vi "VI Data to JSON.vi"(7 "Port number":u16=3363, 8 "error in":errorcluster, 11 "VI Path":path) -> (0 "error out":errorcluster, 3 "JSON string":string)   [LabVIEW 2019]
uses:
  <vilib>/Utility/traverseref.llb/TRef TravTarget.ctl
  <vilib>/Utility/traverseref.llb/VI Scripting - Traverse.lvlib
  <vilib>/Utility/miscctls.llb/LVPositionTypeDef.ctl
  <vilib>/Utility/miscctls.llb/LVMapReplaceAction.ctl
  <vilib>/Utility/miscctls.llb/LVBoundsTypeDef.ctl
  Typedefs/FP Data.ctl
  Typedefs/BD Data.ctl
  Typedefs/VI Data.ctl
  Typedefs/VI Metadata.ctl
  Typedefs/Diagram Group.ctl
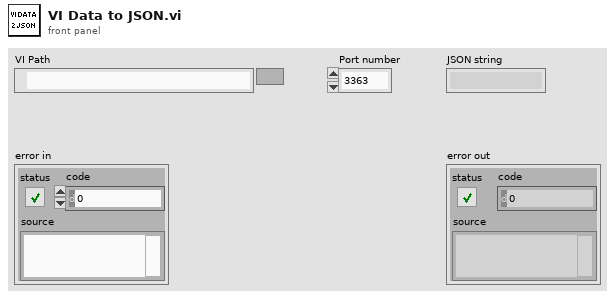
[diagram p1: front panel]
types:
  T1 = typedef "VI Data.ctl" = cluster{"Structure to Diagram":cluster{"UID":i32, "Diagram Group":T2}[], "Diagram to Structure":cluster{"Diagram UID":i32, "Diagram Children":i32[]}[], "FP":T5, "BD":T6, "Metadata":T7}
  T2 = typedef "Diagram Group.ctl" = cluster{"Diagram Data":cluster{"UID":i32, "Diagram Image":string}[], "Position":T3, "Bounds":T4, "Is on TLD?":bool, "Default Frame":u32}
  T3 = typedef "LVPositionTypeDef.ctl" = cluster{"Left":i32, "Top":i32}
  T4 = typedef "LVBoundsTypeDef.ctl" = cluster{"Width":u32, "Height":u32}
  T5 = typedef "FP Data.ctl" = cluster{"Bounds":T4, "Position":T3, "Color":string, "Image":string}
  T6 = typedef "BD Data.ctl" = cluster{"Bounds":T4, "Position":T3, "Color":string, "Image":string}
  T7 = typedef "VI Metadata.ctl" = cluster{"Image":string, "Description":string, "VI Name":string}
  T8 = typedef "imagedata.ctl" = cluster{"image type":i32, "image depth":i32, "image":u8[], "mask":u8[], "colors":u32[], "Rectangle":cluster{"left":i16, "top":i16, "right":i16, "bottom":i16}}
  T9 = typedef "TRef TravTarget.ctl" = enum16{"FP", "BD", "Other"}
  T10 = typedef "LVMapReplaceAction.ctl" = enum32{"Modify Entry only if found", "Add or Modify Entry", "Delete Entry"}
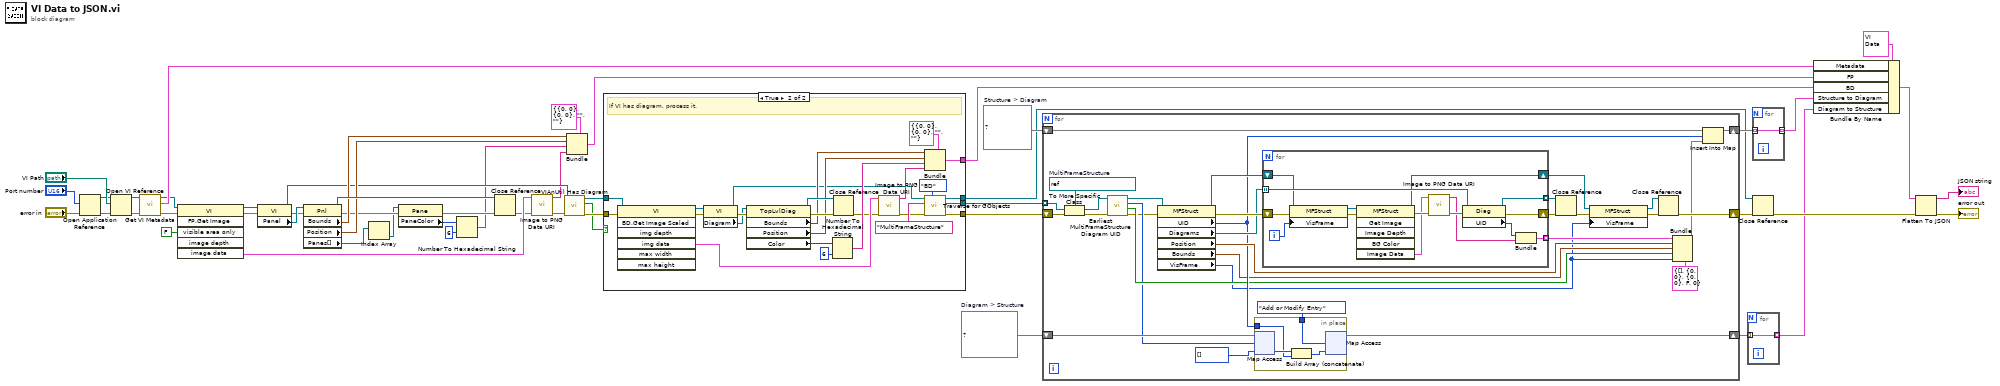
[diagram p0: block diagram]
diagram:
  w41 = map{i32, i32[]} {}  # Diagram > Structure
  w42 = map{i32, T2} {}  # Structure > Diagram
  n1 = Open Application Reference(8:"error in", 10:"Port number") -> (0:w40:errorcluster, 3:w38:refnum<vi>)  [unwired: 2 in]
  n2 = Open VI Reference(application reference (local)=w38, vi path="VI Path", error in (no error)=w40) -> (vi reference=w16:refnum<vi>, error out=w17:errorcluster)  [unwired: 3 in]
  n3 = call "Get VI Metadata.vi"("error in"=w17, "vi reference in"=w16) -> ("error out"=w15:errorcluster, "Metadata"=w14:T7, "vi reference out"=w9:refnum<vi>)  [unwired: 7 in]
  n4 = invoke class="VI" method="FP.Get Image"(reference=w9, error in=w15, "visible area only"=FALSE ("Visible Area Only")) -> (reference out=w34:refnum<vi>, error out=w33:errorcluster, "image data"=w25:T8)  [unwired: 3 in, 3 out]
  n5 = property class="VI"(reference=w34, error in=w33) -> (reference out=w24:refnum<vi>, error out=w35:errorcluster, "Panel"=w36:refnum<vi>)
  n6 = property class="Pnl"(reference=w36, error in=w35) -> (reference out=w32:refnum<vi>, error out=w7:errorcluster, "Bounds"=w31:T4, "Position"=w30:T3, "Panes[]"=w8:refnum<vi>[])
  n7 = Index Array(array=w8) -> (element=w5:refnum<vi>)  [unwired: 1 in]
  n8 = property class="Pane"(reference=w5, error in=w7) -> (error out=w6:errorcluster, "PaneColor"=w3:u32)  [unwired: 1 out]
  n9 = Number To Hexadecimal String(1:i16 6 ("width (-)"), 2:w3) -> (0:w1:string)
  n10 = Close Reference(reference=w32, error in (no error)=w6) -> (error out=w13:errorcluster)
  n11 = call "Image to PNG Data URI.vi"("error in (no error)"=w13, "Image data"=w25) -> ("error out"=w12:errorcluster, "Base64 encoded"=w2:string)  [unwired: 7 in, 1 out]
  n12 = call <vilib>:"VIAnUtil Has Diagram.vi"("error in (no error)"=w12, "VI in"=w24) -> ("error out"=w22:errorcluster, "Has Diag?"=w21:bool, "VI out"=w23:refnum<vi>)  [unwired: 4 in, 3 out]
  n13 = Bundle(cluster=T5 {"Bounds"={"Width"=0, "Height"=0}, "Position"={"Left"=0, "Top"=0}, "Color"="", "Image"=""} ("FP"), "Bounds"=w31, "Position"=w30, "Color"=w1, "Image"=w2) -> (w27:T5)
  n14 = case shown="True" w21 {
    tunnel: [w53 w57] -> w18
    tunnel: [_ w66] -> w28
    tunnel: w23 -> [w52 w63]
    tunnel: w22 -> [w53 w62]
    tunnel: [_ w58] -> w20
    tunnel: [w52 w56] -> w19
    frame False {
      # "If VI does not have diagram (global, control, etc...), skip.\nTool will then show the result as empty block diagram."
    }
    frame True {
      # "If VI has diagram, process it."
      n15 = invoke class="VI" method="BD.Get Image Scaled"(reference=w63, error in=w62) -> (reference out=w77:refnum<vi>, error out=w78:errorcluster, "img data"=w65:T8)  [unwired: 5 in, 4 out]
      n16 = property class="VI"(reference=w77, error in=w78) -> (reference out=w59:refnum<vi>, error out=w76:errorcluster, "Diagram"=w75:refnum<vi>)
      n17 = property class="TopLvlDiag"(reference=w75, error in=w76) -> (reference out=w73:refnum<vi>, error out=w74:errorcluster, "Bounds"=w69:T4, "Position"=w68:T3, "Color"=w71:u32)
      n18 = Number To Hexadecimal String(1:i16 6 ("width (-)"), 2:w71) -> (0:w67:string)
      n19 = Close Reference(reference=w73, error in (no error)=w74) -> (error out=w54:errorcluster)
      n20 = call "Image to PNG Data URI.vi"("error in (no error)"=w54, "Image data"=w65) -> ("error out"=w55:errorcluster, "Base64 encoded"=w64:string)  [unwired: 7 in, 1 out]
      n21 = Bundle(cluster=T6 {"Bounds"={"Width"=0, "Height"=0}, "Position"={"Left"=0, "Top"=0}, "Color"="", "Image"=""} ("BD"), "Bounds"=w69, "Position"=w68, "Color"=w67, "Image"=w64) -> (w66:T6)
      n22 = call <vilib>:"Traverse for GObjects.vi"("Traverse Target"=TRef_TravTarget."BD", "error in (no error)"=w55, "Class Name"="MultiFrameStructure", "VI Refnum"=w59) -> ("error out"=w57:errorcluster, "References"=w58:refnum<vi>[], "dup VI Refnum"=w56:refnum<vi>)  [unwired: 4 in, 1 out]
    }
  }
  n23 = for {
    tunnel: w20 -> [w108] mode=indexing
    shift-right: [w103] -> w49
    shift-left: w42 -> [w104]
    shift-right: [w100] -> w50
    shift-left: w18 -> [w109]
    shift-right: [w93] -> w47
    shift-left: w41 -> [w94]
    w107 = refnum<vi> refnum  # MultiFrameStructure
    n24 = To More Specific Class(target class=w107, reference=w108, error in=w109) -> (specific class reference=w84:refnum<vi>, error out=w86:errorcluster)
    n25 = call "Earliest MultiFrameStructure Diagram UID.vi"("error in (no error)"=w86, "MFS ref in"=w84) -> ("error out"=w85:errorcluster, "TLD?"=w88:bool, "UID"=w87:i32, "MFS ref out"=w83:refnum<vi>)  [unwired: 6 in]
    n26 = property class="MFStruct"(reference=w83, error in=w85) -> (reference out=w99:refnum<vi>, error out=w106:errorcluster, "UID"=w91:i32, "Diagrams"=w105:refnum<vi>[], "Position"=w98:T3, "Bounds"=w89:T4, "VisFrame"=w79:u32)
    n27 = in-place {
      in-place-border: LVMapReplaceAction."Add or Modify Entry" ("Replace Action") -> [w111]
      in-place-border: w91 -> [w110]
      n28 = in-place-map #1(w94, w87, i32[] [] ("output cluster")) -> (w113:i32[])  [unwired: 1 out]
      n29 = Build Array (concatenate)(w113, w110) -> (w112:i32[])
      n30 = in-place-map #1(w112, w111) -> (w93:map{i32, i32[]})  [unwired: 2 out]
    }
    n31 = for {
      tunnel: w105 -> [w128] mode=indexing
      tunnel: [w119] -> w97 mode=indexing
      shift-right: [w127] -> w102
      shift-left: w106 -> [w125]
      tunnel: [w126] -> w101 mode=indexing
      shift-right: [w114] -> w81
      shift-left: w99 -> [w124]
      i -> [w123]
      n32 = property class="MFStruct"(reference=w124, error in=w125, "VisFrame"=w123) -> (reference out=w121:refnum<vi>, error out=w122:errorcluster)
      n33 = invoke class="MFStruct" method="Get Image"(reference=w121, error in=w122) -> (reference out=w114:refnum<vi>, error out=w118:errorcluster, "Image Data"=w116:T8)  [unwired: 4 in, 3 out]
      n34 = call "Image to PNG Data URI.vi"("error in (no error)"=w118, "Image data"=w116) -> ("error out"=w117:errorcluster, "Base64 encoded"=w115:string)  [unwired: 7 in, 1 out]
      n35 = property class="Diag"(reference=w128, error in=w117) -> (reference out=w126:refnum<vi>, error out=w127:errorcluster, "UID"=w120:i32)
      n36 = Bundle("UID"=w120, "Base64 encoded"=w115) -> (w119:cluster{"UID":i32, "Base64 encoded":string})  [unwired: 1 in]
    }
    n37 = Close Reference(reference=w101, error in (no error)=w102) -> (error out=w82:errorcluster)
    n38 = property class="MFStruct"(reference=w81, "VisFrame"=w79) -> (reference out=w80:refnum<vi>)  [unwired: 1 in, 1 out]
    n39 = Close Reference(reference=w80, error in (no error)=w82) -> (error out=w100:errorcluster)
    n40 = Bundle(cluster=T2 {"Diagram Data"=[], "Position"={"Left"=0, "Top"=0}, "Bounds"={"Width"=0, "Height"=0}, "Is on TLD?"=FALSE, "Default Frame"=0} ("Diagram Group"), "Diagram Data"=w97, "Position"=w98, "Bounds"=w89, "Is on TLD?"=w88, "Default Frame"=w79) -> (w96:T2)
    n41 = Insert Into Map(map in=w104, key=w91, value=w96) -> (map out=w103:map{i32, T2})  [unwired: 2 out]
  }
  n42 = for {
    tunnel: w47 -> [w129] mode=indexing
    tunnel: [w129] -> w43 mode=indexing
  }
  n43 = for {
    tunnel: w49 -> [w130] mode=indexing
    tunnel: [w130] -> w44 mode=indexing
  }
  n44 = Close Reference(reference=w19, error in (no error)=w50) -> (error out=w46:errorcluster)
  n45 = Bundle By Name(cluster=T1 {"Structure to Diagram"=[], "Diagram to Structure"=[], "FP"={"Bounds"={"Width"=0, "Height"=0}, "Position"={"Left"=0, "Top"=0}, "Color"="", "Image"=""}, "BD"={"Bounds"={"Width"=0, "Height"=0}, "Position"={"Left"=0, "Top"=0}, "Color"="", "Image"=""}, "Metadata"={"Image"="", "Description"="", "VI Name"=""}}, "Metadata"=w14, "FP"=w27, "BD"=w28, "Structure to Diagram"=w44, "Diagram to Structure"=w43) -> (w48:T1)
  n46 = Flatten To JSON(anything=w48, error in (no error)=w46) -> (JSON string=→"JSON string":string, 11:→"error out":errorcluster)  [unwired: 1 in]
